vi "Create Menus.vi"(6 "menu options":cluster{"open":bool, "save":bool, "view":bool}={"open"=TRUE, "save"=FALSE, "view"=FALSE}, 8 "error in (no error)":errorcluster, 11 "Application Data in":T1={"Item Tree Control"=refnum, "Top-Level VI"=refnum, "menu reference"=refnum, "queue"=refnum, "Stop Pointer"=refnum, "Buffer Variant"=variant, "server ID"=refnum, "framework tag"="", "Values"=refnum, "Hex"=refnum, "ASCII"=refnum, "lines visible"=0, "values padding"=0, "current buffer data"={"decimation"=0, "avg bandwidth"=0.0, "channels"=[], "byte order"=enum."little-endian", "buffer descriptor"={"buffer type"=enum."Engine", "plugin id"=0, "group id"=0, "transfer id"=0, "offset"=0, "length"=0}, "values channels"={"index"=0, "count"=0, "engine offset"=0}, "select start offset"=18446744073709551615, "select end offset"=0, "channel index"=-1}, "Framework Configuration"=refnum} {"current buffer data"."channels"."configuration"."string offset" format="%d bytes"; "current buffer data"."avg bandwidth" format="%.0g bytes"}) -> (0 "error out":errorcluster, 3 "Application Data out":T1={"Item Tree Control"=refnum, "Top-Level VI"=refnum, "menu reference"=refnum, "queue"=refnum, "Stop Pointer"=refnum, "Buffer Variant"=variant, "server ID"=refnum, "framework tag"="", "Values"=refnum, "Hex"=refnum, "ASCII"=refnum, "lines visible"=0, "values padding"=0, "current buffer data"={"decimation"=0, "avg bandwidth"=0.0, "channels"=[], "byte order"=enum."little-endian", "buffer descriptor"={"buffer type"=enum."Engine", "plugin id"=0, "group id"=0, "transfer id"=0, "offset"=0, "length"=0}, "values channels"={"index"=0, "count"=0, "engine offset"=0}, "select start offset"=18446744073709551615, "select end offset"=0, "channel index"=-1}, "Framework Configuration"=refnum} {"current buffer data"."channels"."configuration"."string offset" format="%d bytes"; "current buffer data"."avg bandwidth" format="%.0g bytes"})   [LabVIEW 2021, in "DSF Core.lvlib"]
uses:
  DSF Core.lvlib
  Application Data.ctl
  <vilib>/NI/Memory Manager/Classes/Pointer/Pointer.lvclass
  Classes/Configuration/Core/Framework/Framework Configuration.lvclass
  Buffer Reader/Queue Data.ctl
  Buffer Reader/Buffer Data.ctl
  Classes/Configuration/Core/Transfer/Channel Configuration.ctl
  Typedefs/Core Channel Configuration.ctl
  Typedefs/DSF Data Type.ctl
  Typedefs/DSF Settings Info.ctl
  Typedefs/DSF Byte Order.ctl
  Classes/Thread/Data Server/DSF Buffer Subset Descriptor.ctl
  Typedefs/DSF Buffer Type.ctl
  Values Channels.ctl
  Classes/Configuration/Core/Channel/Channel Configuration.lvclass
  Classes/Configuration/Core/Transfer/Transfer Configuration.lvclass
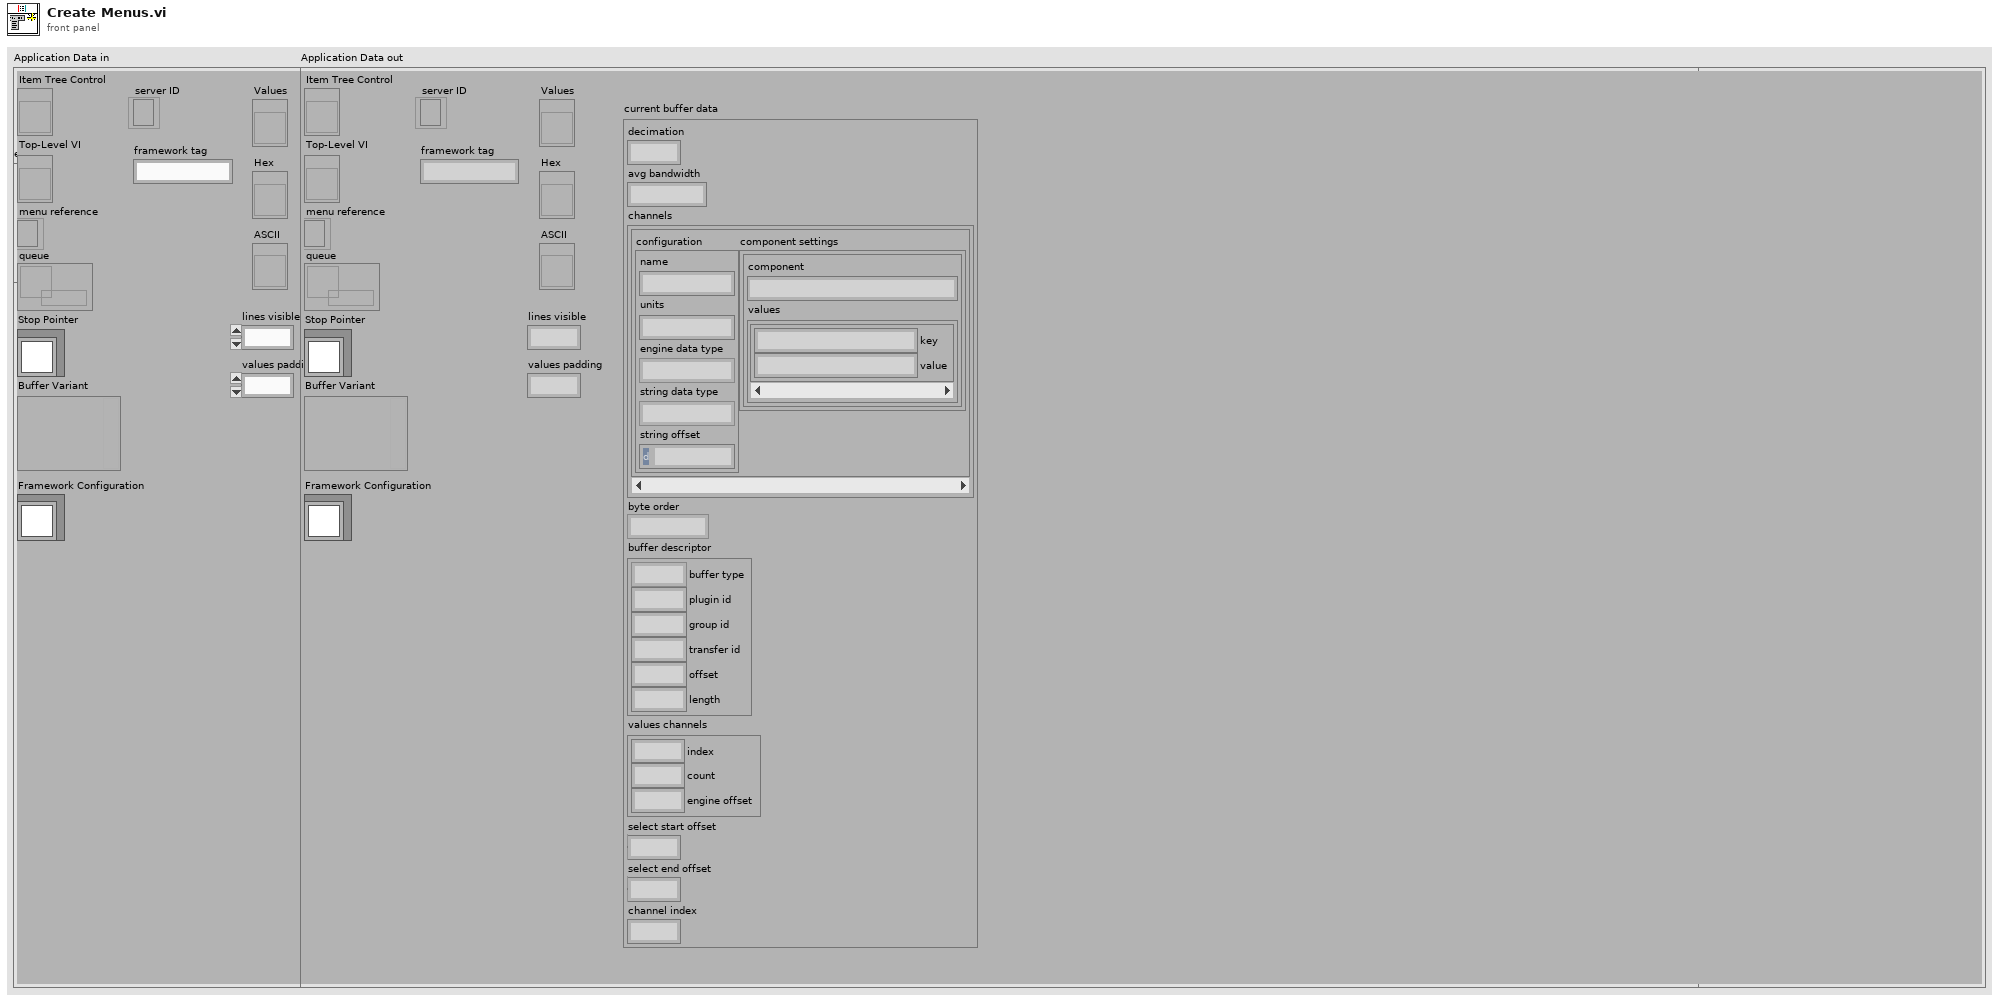
[diagram p1: front panel]
types:
  T1 = typedef "DSF Core.lvlib/Application Data.ctl" = cluster{"Item Tree Control":refnum<vi>, "Top-Level VI":refnum<vi>, "menu reference":refnum<k9>, "queue":refnum<queue>, "Stop Pointer":refnum<class "Pointer.lvclass">, "Buffer Variant":variant, "server ID":refnum<k5>, "framework tag":string, "Values":refnum<vi>, "Hex":refnum<vi>, "ASCII":refnum<vi>, "lines visible":i32, "values padding":i32, "current buffer data":T2, "Framework Configuration":refnum<class "Framework Configuration.lvclass">}
  T2 = typedef "DSF Core.lvlib/Buffer Data.ctl" = cluster{"decimation":u64, "avg bandwidth":dbl, "channels":T3[], "byte order":T7, "buffer descriptor":T8, "values channels":T10, "select start offset":u64, "select end offset":u64, "channel index":i32}
  T3 = typedef "DSF Core.lvlib/Transfer Configuration.lvclass/Channel Configuration.ctl" = cluster{"configuration":T4, "component settings":T6[]}
  T4 = typedef "DSF Core.lvlib/Channel Configuration.lvclass/Core Channel Configuration.ctl" = cluster{"name":string, "units":string, "engine data type":T5, "string data type":T5, "string offset":u64}
  T5 = typedef "DSF Core.lvlib/DSF Data Type.ctl" = enum8{"Bool", "SGL", "DBL", "I8", "I16", "I32", "I64", "U8", "U16", "U32", "U64"}
  T6 = typedef "DSF Core.lvlib/DSF Settings Info.ctl" = cluster{"component":string, "values":cluster{"key":string, "value":string}[]}
  T7 = typedef "DSF Core.lvlib/DSF Byte Order.ctl" = enum8{"big-endian", "little-endian"}
  T8 = typedef "DSF Core.lvlib/DSF Buffer Subset Descriptor.ctl" = cluster{"buffer type":T9, "plugin id":i32, "group id":i32, "transfer id":i32, "offset":u64, "length":i64}
  T9 = typedef "DSF Core.lvlib/DSF Buffer Type.ctl" = enum16{"Engine", "String"}
  T10 = typedef "DSF Core.lvlib/Values Channels.ctl" = cluster{"index":i32, "count":i32, "engine offset":u64}
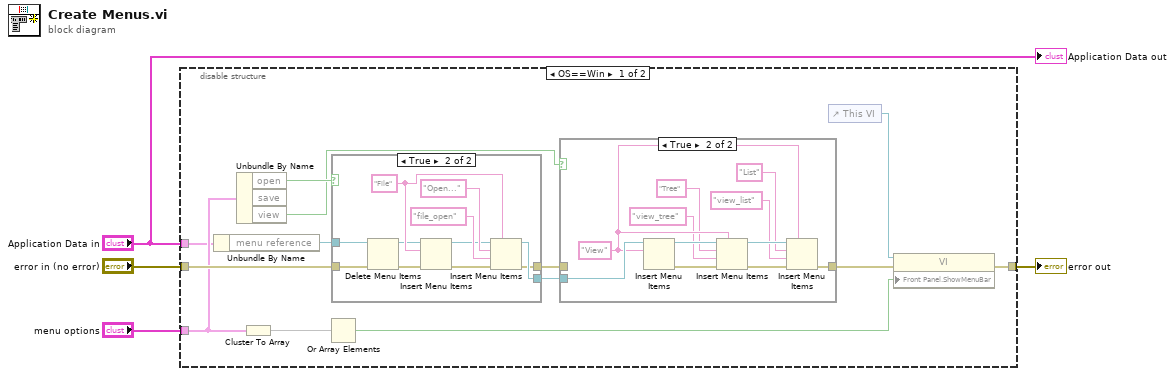
[diagram p0: block diagram]
diagram:
  n1 = disable-structure shown="OS==Win" {
    disable-tunnel: "error in (no error)" -> [w17 w43]
    disable-tunnel: "menu options" -> [w12 _]
    disable-tunnel: [w7 w43] -> w2
    disable-tunnel: "Application Data in" -> [w6 _]
    frame condition #0 {
      n2 = Unbundle By Name(w6) -> ("menu reference"=w5:refnum<k9>)
      n3 = Unbundle By Name(w12) -> ("open"=w15:bool, "view"=w14:bool)  [unwired: 1 out]
      n4 = Cluster To Array(cluster=w12) -> (array=w11:bool[])
      n5 = Or Array Elements(Boolean array=w11) -> (logical OR=w9:bool)
      n6 = case shown="True" w15 {
        tunnel: w17 -> [w30 w42]
        tunnel: [w31 w40] -> w16
        tunnel: w5 -> [w31 w33]
        tunnel: [w30 w32] -> w13
        frame False {
        }
        frame True {
          w37 = "File" ("item names")
          n7 = Delete Menu Items(6:w42, 9:w33) -> (0:w41:errorcluster, 3:w34:refnum<k9>)  [unwired: 2 in]
          n8 = Insert Menu Items(6:w41, 8:w37, 9:w34) -> (0:w35:errorcluster, 3:w36:refnum<k9>)  [unwired: 3 in, 1 out]
          n9 = Insert Menu Items(5:w37, 6:w35, 7:"file_open" ("item tags"), 8:"Open..." ("item names"), 9:w36) -> (0:w32:errorcluster, 3:w40:refnum<k9>)  [unwired: 1 in, 1 out]
        }
      }
      n10 = case shown="True" w14 {
        tunnel: [w18 w29] -> w8
        tunnel: w16 -> [_ w28]
        tunnel: w13 -> [w18 _]
        frame False {
        }
        frame True {
          w26 = "View" ("item names")
          n11 = Insert Menu Items(8:w26, 9:w28) -> (0:w22:errorcluster, 3:w21:refnum<k9>)  [unwired: 4 in, 1 out]
          n12 = Insert Menu Items(5:w26, 6:w22, 7:"view_tree" ("item tags"), 8:"Tree" ("item names"), 9:w21) -> (0:w27:errorcluster, 3:w25:refnum<k9>)  [unwired: 1 in, 1 out]
          n13 = Insert Menu Items(5:w26, 6:w27, 7:"view_list" ("item tags"), 8:"List" ("item names"), 9:w25) -> (0:w29:errorcluster)  [unwired: 1 in, 2 out]
        }
      }
      n14 = control-ref of="This VI"() -> (w10:refnum<vi>)
      n15 = property class="VI"(reference=w10, error in=w8, "Front Panel.ShowMenuBar"=w9) -> (error out=w7:errorcluster)  [unwired: 1 out]
    }
    frame condition #1 (active) {
    }
  }
  "error out" <- w2
  "Application Data out" <- "Application Data in"
